vi "HackRF_SetFreq_Carrier.vi"(8 "error in (no error)":errorcluster, 10 "CarrierFreqHz":dbl format="%#_6p", 11 "HackRF_In":T1) -> (0 "error out":errorcluster, 3 "HackRF_Out":T1)   [LabVIEW 2016]
uses:
  HackRF_Ref.ctl
  C:/Program Files/HackRF/labview/NetHackrf.dll
  NetHackrf.dll
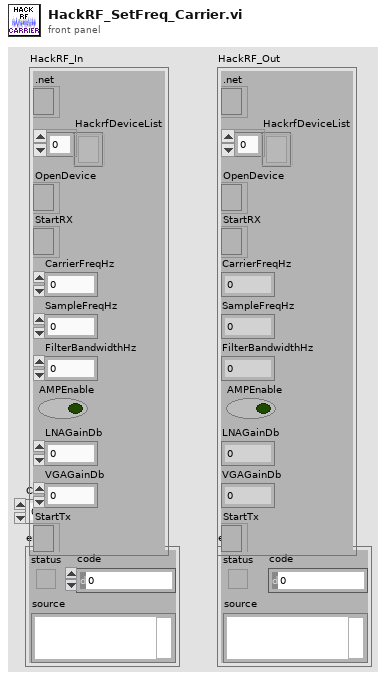
[diagram p1: front panel]
types:
  T1 = typedef "HackRF_Ref.ctl" = cluster{".net":refnum<k24>, "HackrfDeviceList":refnum<k24>[], "OpenDevice":refnum<k24>, "StartRX":refnum<k24>, "CarrierFreqHz":dbl, "SampleFreqHz":dbl, "FilterBandwidthHz":dbl, "AMPEnable":bool, "LNAGainDb":dbl, "VGAGainDb":dbl, "StartTx":refnum<k24>}
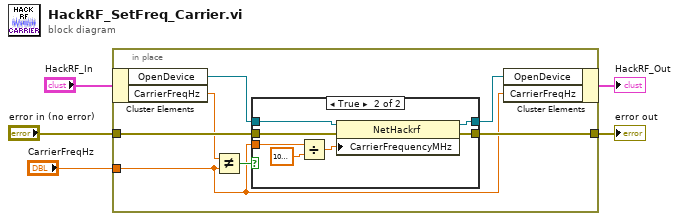
[diagram p0: block diagram]
diagram:
  n1 = in-place {
    in-place-border: [w10] -> w5
    in-place-border: "error in (no error)" -> [w9]
    in-place-border: "CarrierFreqHz" -> [w6]
    n2 = in-place-cluster #1("HackRF_In") -> ("OpenDevice"=w12:refnum<k24>, "CarrierFreqHz"=w8:dbl)
    n3 = Not Equal?(x=w8, y=w6) -> (x != y?=w7:bool)
    n4 = case shown="True" w7 {
      tunnel: w12 -> [w13 w21]
      tunnel: [w13 w20] -> w11
      tunnel: [w14 w19] -> w10
      tunnel: w9 -> [w14 w18]
      tunnel: w6 -> [_ w17]
      frame False {
      }
      frame True {
        n5 = Divide(x=w17, y=1000000.0) -> (x/y=w15:dbl)
        n6 = property class="NetHackrf"(reference=w21, error in=w18, "CarrierFrequencyMHz"=w15) -> (reference out=w20:refnum<k24>, error out=w19:errorcluster)
      }
    }
    n7 = in-place-cluster #1("OpenDevice"=w11, "CarrierFreqHz"=w6) -> (→"HackRF_Out":T1)
  }
  "error out" <- w5
